vi "Set AO Chan.vi"(8 "error in (no error)":errorcluster caption="错误输入（无错误）", 10 "AO设置.DAQmx物理通道":tag, 11 "DAQ 输入":refnum<class "DAQ.lvclass">) -> (0 "error out":errorcluster caption="错误输出", 3 "DAQ 输出":refnum<class "DAQ.lvclass">)   [LabVIEW 2017, in "DAQ.lvlib" / "DAQ.lvclass"]
uses:
  DAQ.lvclass
  E:/Program Files (x86)/National Instruments/LabVIEW 2017/vi.lib/ActorFramework/Actor/Actor.lvclass
  DAQ.lvclass/DAQ.ctl
  <vilib>/ActorFramework/Actor/Actor.lvclass/Actor.ctl
  <vilib>/ActorFramework/Message Enqueuer/Message Enqueuer.lvclass/Message Enqueuer.ctl
  <vilib>/ActorFramework/Message Enqueuer/Enqueue.vi
  E:/Program Files (x86)/National Instruments/LabVIEW 2017/vi.lib/ActorFramework/Message/Message.lvclass
  <vilib>/ActorFramework/Message Priority Queue/Priority Enqueue.vi
  <vilib>/ActorFramework/Actor/Actor.lvclass
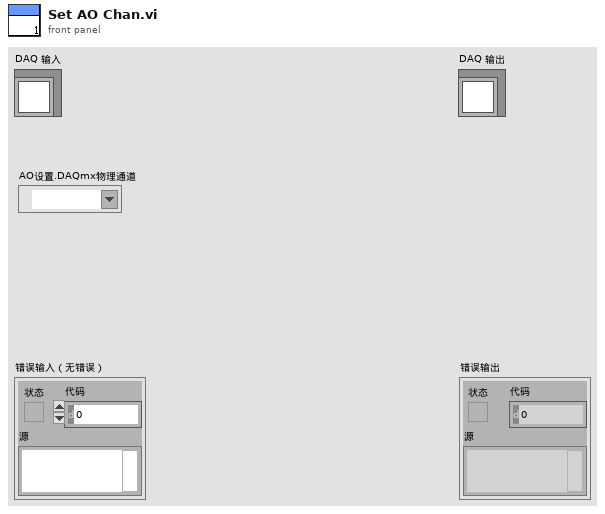
[diagram p1: front panel]
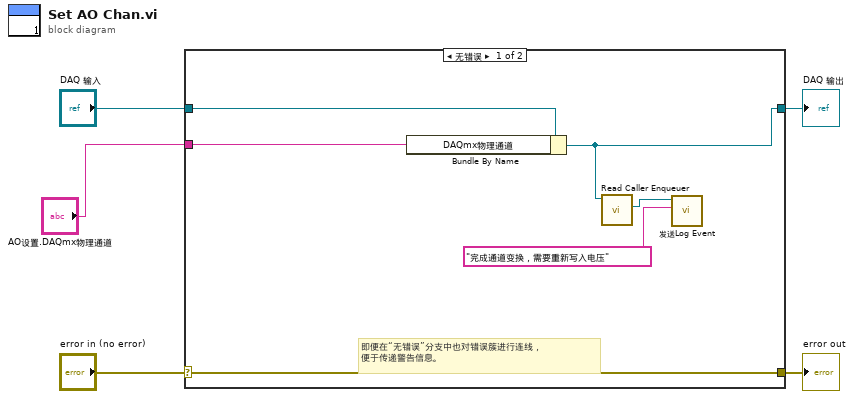
[diagram p0: block diagram]
diagram:
  n1 = case shown="无错误" "error in (no error)" {
    selector: "error in (no error)" -> [w11 w13]
    tunnel: [w11 w13] -> w4
    tunnel: [w8 w12] -> w2
    tunnel: "DAQ 输入" -> [w10 w12]
    tunnel: "AO设置.DAQmx物理通道" -> [w9 _]
    frame No Error {
      # "即便在“无错误”分支中也对错误簇进行连线，\n便于传递警告信息。"
      n2 = Bundle By Name(cluster=w10, "DAQmx物理通道"=w9) -> (w8:refnum<class "DAQ.lvclass">)
      n3 = call <vilib>:"Read Caller Enqueuer.vi"("Actor"=w8) -> ("Caller Enqueuer"=w7:refnum<class "Message Enqueuer.lvclass">)  [unwired: 10 in]
      n4 = call "发送Log Event.vi"("事件文本"="完成通道变换，需要重新写入电压", "Message Enqueuer"=w7) -> ()  [unwired: 8 in, 2 out]
    }
    frame Error {
    }
  }
  "error out" <- w4
  "DAQ 输出" <- w2
